vi "Run.vi"(9 "Messages":refnum<event-registration>, 10 "Message-Enqueue Refs":T1, 11 "Actor in":refnum<class "Actor.lvclass">) -> (0 "error out":errorcluster, 3 "Actor out":refnum<class "Actor.lvclass">)   [LabVIEW 2018, in "Actor.lvclass"]
uses:
  Actor.lvclass
  Message-Enqueuer References.ctl
  Stop.ctl
  Launch.ctl
  Did Initialize.ctl
  <vilib>/Utility/error.llb/Error Cluster From Error Code.vi
  <vilib>/ErrorRing/Error Ring.xnode
panel:
  in  "Simulate Error":bool
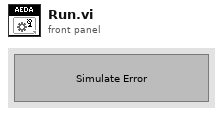
[diagram p1: front panel]
types:
  T1 = typedef "Actor.lvclass/Message-Enqueuer References.ctl" = cluster{"Stop":refnum<user-event>, "Launch":refnum<user-event>, "Did Initialize":refnum<user-event>}
  T2 = cluster{"Messages":refnum<event-registration>, "Messages":refnum<event-registration>}
  T3 = typedef "Actor.lvclass/Stop.ctl" = cluster{"Type":enum16{"Normal", "Emergency"}}
  T4 = typedef "Actor.lvclass/Did Initialize.ctl" = cluster{"State":refnum<class "Actor.lvclass">}
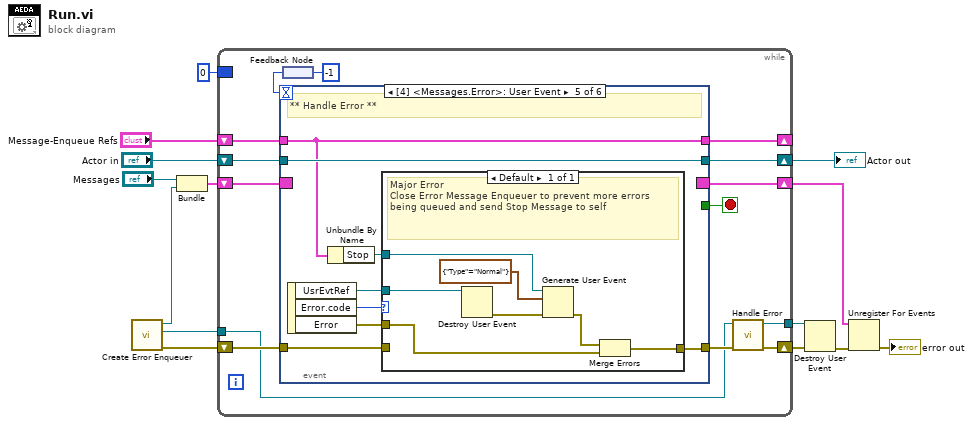
[diagram p0: block diagram]
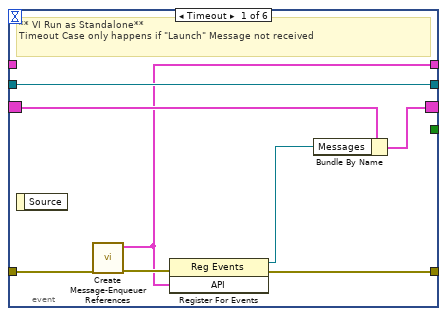
[diagram p2: hidden frame]
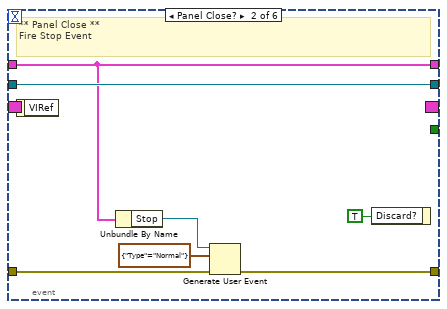
[diagram p3: hidden frame]
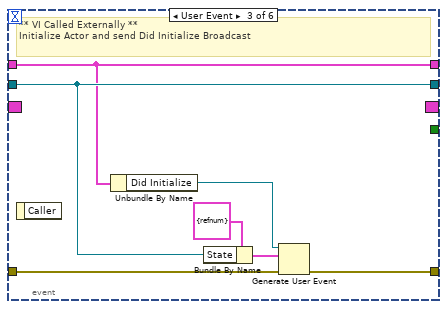
[diagram p4: hidden frame]
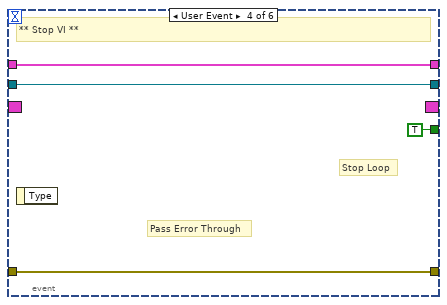
[diagram p5: hidden frame]
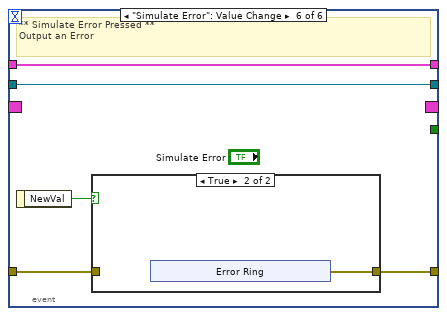
[diagram p6: hidden frame]
diagram:
  n1 = call "Create Error Enqueuer.vi"() -> ("error out"=w11:errorcluster, "Error Enqueuer"=w5:refnum<user-event>, "Messages"=w8:refnum<event-registration>)  [unwired: 9 in]
  n2 = Bundle("Messages"="Messages", "Messages"=w8) -> (w7:T2)  [unwired: 1 in]
  n3 = while {
    shift-right: [w26] -> w13
    shift-left: "Actor in" -> [w28]
    shift-right: [w23] -> w4
    shift-left: w11 -> [w27]
    shift-right: [w19] -> w1
    shift-left: w7 -> [w18]
    shift-right: [w17] -> _
    shift-left: "Message-Enqueue Refs" -> [w22]
    border: 0 -> [_]
    tunnel: w5 -> [w16]
    tunnel: [w15] -> w3
    stop <- w25 stop-if-true
    n4 = feedback-in #1(-1) -> ()
    n5 = feedback #1() -> (w20:i32)
    n6 = event shown="[4] <Messages.Error>: User Event" {
      selector: w18 -> [w32 _ _ _ _ _]
      dyn-events: [w30 _ _ _ _ _] -> w19
      timeout: w20 -> [_ _ _ _ _ _]
      tunnel: w28 -> [w33 w43 w47 w54 w62 w73]
      tunnel: w27 -> [w36 w41 w44 w53 w59 w71]
      tunnel: [w33 w43 w47 w54 w62 w73] -> w26
      tunnel: [w34 w40 w46 w53 w57 w70] -> w24
      tunnel: [_ _ _ TRUE _ _] -> w25
      tunnel: w22 -> [_ w37 w45 w51 w56 w74]
      tunnel: [w29 w37 w45 w51 w56 w74] -> w17
      event Timeout {
        # "** VI Run as Standalone**\nTimeout Case only happens if \"Launch\" Message not received"
        n7 = event-data() -> ()  [unwired: 1 in, 1 out]
        n8 = call "Create Message-Enqueuer References.vi"("error in (no error)"=w36) -> ("error out"=w35:errorcluster, "API"=w29:T1)  [unwired: 9 in]
        n9 = register-events(error in=w35, w29) -> (reference out=w31:refnum<event-registration>, error out=w34:errorcluster)  [unwired: 1 in]
        n10 = Bundle By Name(cluster=w32, "Messages"=w31) -> (w30:T2)
      }
      event Panel Close? {
        # "** Panel Close **\nFire Stop Event"
        n11 = event-data() -> ()  [unwired: 1 in, 1 out]
        n12 = Unbundle By Name(w37) -> ("Stop"=w39:refnum<user-event>)
        n13 = Generate User Event(user event=w39, event data cluster=T3 {"Type"=enum."Normal"} ("event data"), error in=w41) -> (error out=w40:errorcluster)  [unwired: 1 in, 1 out]
        n14 = event-data("Discard?"=TRUE) -> ()  [unwired: 1 in, 1 out]
      }
      event User Event {
        # "** VI Called Externally **\nInitialize Actor and send Did Initialize Broadcast"
        n15 = event-data() -> ()  [unwired: 1 in, 1 out]
        n16 = Unbundle By Name(w45) -> ("Did Initialize"=w50:refnum<user-event>)
        n17 = Bundle By Name(cluster=T4 {"State"=refnum} ("Did Initialize"), "State"=w47) -> (w48:T4)
        n18 = Generate User Event(user event=w50, event data cluster=w48, error in=w44) -> (error out=w46:errorcluster)  [unwired: 1 in, 1 out]
      }
      event User Event {
        # "Stop Loop"
        # "Pass Error Through"
        # "** Stop VI **"
        n19 = event-data() -> ()  [unwired: 1 in, 1 out]
      }
      event User Event {
        # "** Handle Error **"
        n20 = event-data() -> ("UsrEvtRef"=w55:refnum<user-event>, "Error.code"=w61:i32, "Error"=w60:errorcluster)  [unwired: 1 in]
        n21 = Unbundle By Name(w56) -> ("Stop"=w58:refnum<user-event>)
        n22 = case shown="Default" w61 {
          tunnel: w60 -> [w67]
          tunnel: w59 -> [_]
          tunnel: w58 -> [w69]
          tunnel: [w66] -> w57
          tunnel: w55 -> [w63]
          frame Default {
            # "Major Error\nClose Error Message Enqueuer to prevent more errors being queued and send Stop Message to self"
            n23 = Destroy User Event(user event=w63) -> (error out=w68:errorcluster)  [unwired: 1 in]
            n24 = Generate User Event(user event=w69, event data cluster=T3 {"Type"=enum."Normal"} ("event data"), error in=w68) -> (error out=w65:errorcluster)  [unwired: 1 in, 1 out]
            n25 = Merge Errors(w65, w67) -> (w66:errorcluster)
          }
        }
      }
      event "Simulate Error": Value Change {
        # "** Simulate Error Pressed **\nOutput an Error"
        n26 = event-data() -> ("NewVal"=w72:bool)  [unwired: 1 in]
        n27 = case shown="True" w72 {
          tunnel: w71 -> [w75 _]
          tunnel: [w75 w76] -> w70
          frame False {
          }
          frame True {
            n28 = xnode "Error Ring"() -> ("error out"=w76:errorcluster)
          }
        }
      }
    }
    n29 = call "Handle Error.vi"("error in (no error)"=w24, "Error Enqueuer in"=w16) -> ("error out"=w23:errorcluster, "Error Enqueuer out"=w15:refnum<user-event>)  [unwired: 8 in]
  }
  "Actor out" <- w13
  n30 = Destroy User Event(user event=w3, error in=w4) -> (error out=w2:errorcluster)
  n31 = Unregister For Events(event registration refnum=w1, error in=w2) -> (error out=→"error out":errorcluster)
